vi "ziModGetCounterData.vi"(8 "Error In":errorcluster, 10 "ModResults":T3, 11 "ModHandle In":T6 {"ModHandle" format="0x%08x"; "Conn" format="0x%08x"}) -> (0 "Error Out":errorcluster, 2 "ModCntData":T2[](array[typedef]), 3 "ModHandle Out":T6 {"ModHandle" format="0x%08x"; "Conn" format="0x%08x"})   [LabVIEW 2009, in "Zurich Instruments LabOne.lvlib"]
doc: "Use this vi to get Counter Data from a ModResult returned from ziModGetNextNode.vi. It returns an array of Counter Data."
uses:
  <instrlib>/Zurich Instruments LabOne/Zurich Instruments LabOne.lvlib
  <instrlib>/Zurich Instruments LabOne/Public/Modules/ziTypeModHandle.ctl
  <instrlib>/Zurich Instruments LabOne/Public/Modules/ziTypeModResults.ctl
  <instrlib>/Zurich Instruments LabOne/Public/Data/ziTypePollType.ctl
  <instrlib>/Zurich Instruments LabOne/Public/Modules/ziTypeModGenericHeader.ctl
  <instrlib>/Zurich Instruments LabOne/Public/Data/ziTypeCounterSample.ctl
  <instrlib>/Zurich Instruments LabOne/Public/Data/ziTypeCounterSampleGrid.ctl
  <instrlib>/Zurich Instruments LabOne/Private/ziLV32.dll
panel:
  out "ModCntDataGrid":T1[](array[typedef])
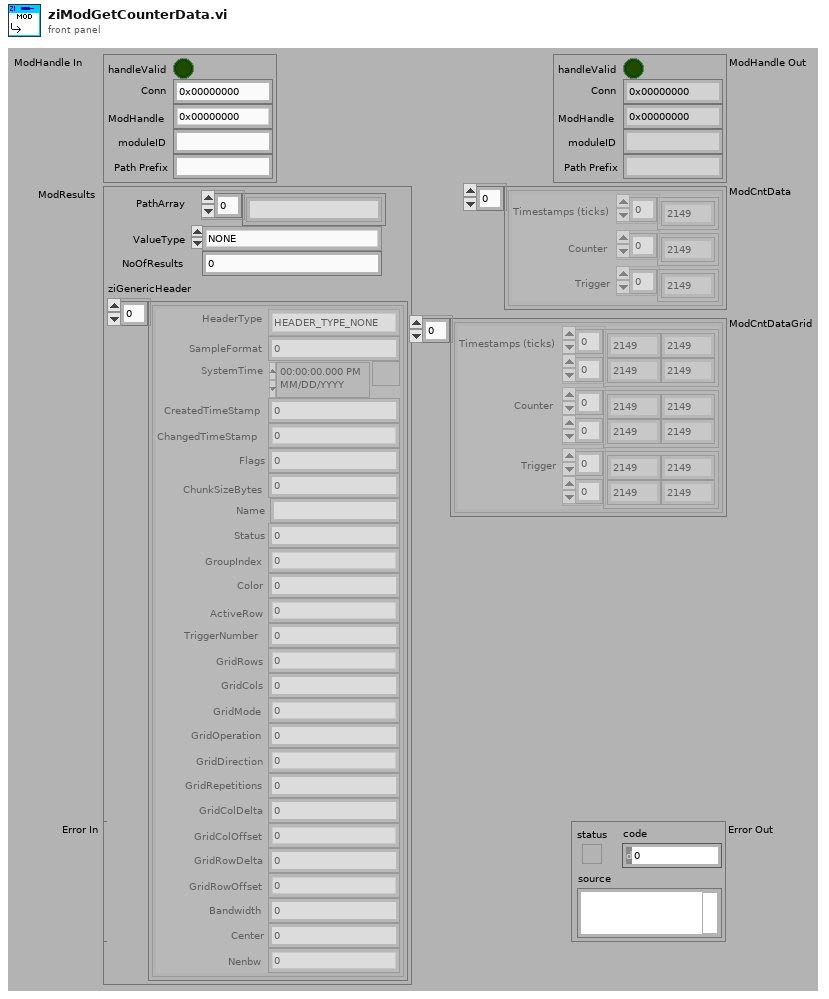
[diagram p1: front panel]
types:
  T1 = typedef "Zurich Instruments LabOne.lvlib/ziTypeCounterSampleGrid.ctl" = cluster{"Timestamps (ticks)":u64[][], "Counter":i32[][], "Trigger":u32[][]}
  T2 = typedef "Zurich Instruments LabOne.lvlib/ziTypeCounterSample.ctl" = cluster{"Timestamps (ticks)":u64[], "Counter":i32[], "Trigger":u32[]}
  T3 = typedef "Zurich Instruments LabOne.lvlib/ziTypeModResults.ctl" = cluster{"PathArray":string[], "ValueType":T4, "NoOfResults":u64, "ziGenericHeader":T5[]}
  T4 = typedef "Zurich Instruments LabOne.lvlib/ziTypePollType.ctl" = enum16{"NONE", "DOUBLE_DATA", "INTEGER_DATA", "DEMOD_SAMPLE", "SCOPE_WAVE_HF2", "AUXIN_SAMPLE", "DIO_SAMPLE", "BYTE_ARRAY", "PWA_WAVE", "9", "10", "11", "12", "13", "14", "15", "TREE_CHANGE_DEPRI", "17", "ERROR", "19", "20", "21", "22", "23", "24", "25", "26", "27", "28", "29", "30", "31", "DOUBLE_DATA_TS", "INTEGER_DATA_TS", "34", "SCOPE_WAVE", "SCOPE_WAVE_EX", "37", "BYTE_ARRAY_TS", "39", "40", "41", "42", "43", "44", "45", "CNT_DATA", "47", "TREE_CHANGE", "49", "50", "51", "52", "53", "54", "55", "56", "57", "58", "59", "60", "61", "62", "63", "SWEEPER_DATA", "SPECTRUM_DATA", "ADVISOR_DATA", "VECTOR_DATA", "IMP_DATA"}
  T5 = typedef "Zurich Instruments LabOne.lvlib/ziTypeModGenericHeader.ctl" = cluster{"HeaderType":enum8{"HEADER_TYPE_NONE", "HEADER_TYPE_SWTRIGGER", "HEADER_TYPE_SWEEPER"}, "SampleFormat":u8, "SystemTime":timestamp, "CreatedTimeStamp":u64, "ChangedTimeStamp":u64, "Flags":u32, "ChunkSizeBytes":u64, "Name":string, "Status":u32, "GroupIndex":u32, "Color":u32, "ActiveRow":u32, "TriggerNumber":u64, "GridRows":u32, "GridCols":u32, "GridMode":u32, "GridOperation":u32, "GridDirection":u32, "GridRepetitions":u32, "GridColDelta":dbl, "GridColOffset":dbl, "GridRowDelta":dbl, "GridRowOffset":dbl, "Bandwidth":dbl, "Center":dbl, "Nenbw":dbl}
  T6 = typedef "Zurich Instruments LabOne.lvlib/ziTypeModHandle.ctl" = cluster{"handleValid":bool, "Conn":u64, "ModHandle":u64, "moduleID":string, "Path Prefix":string}
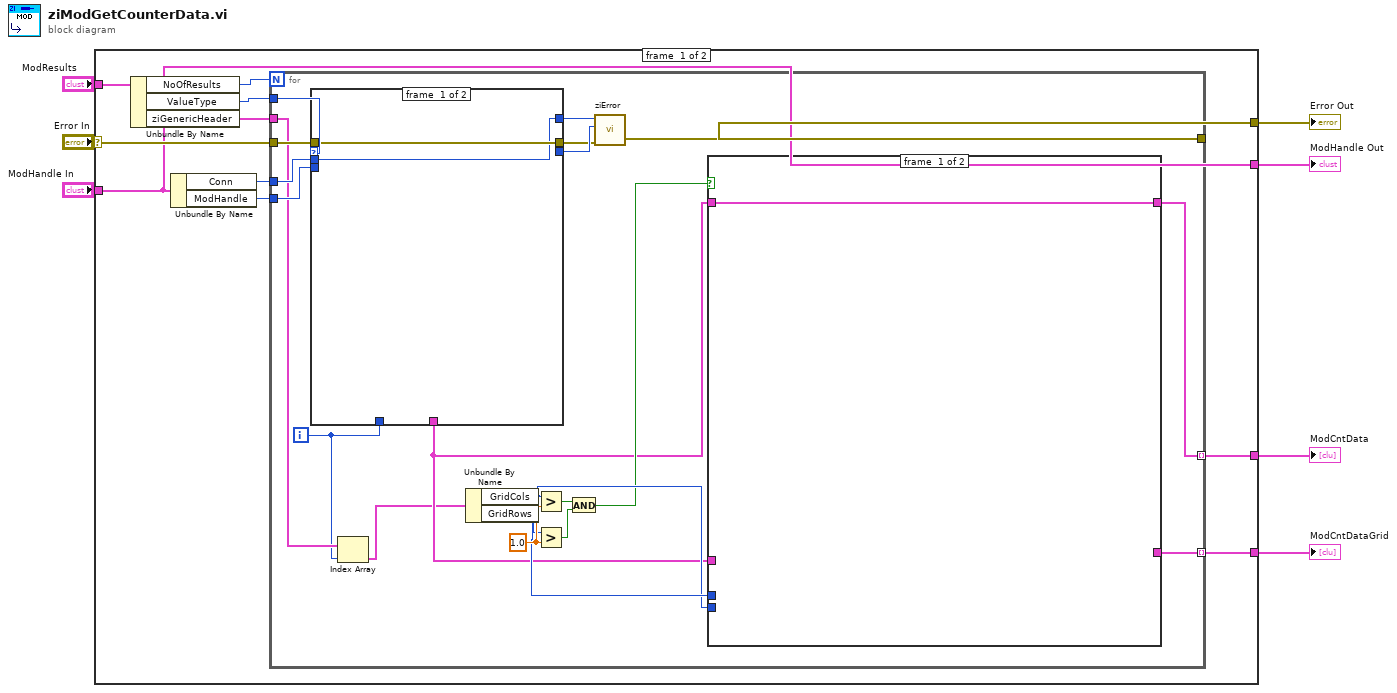
[diagram p0: block diagram]
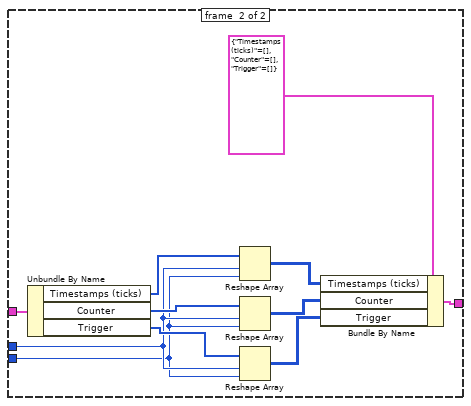
[diagram p2: hidden frame]
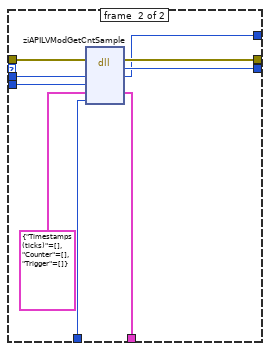
[diagram p3: hidden frame]
diagram:
  n1 = case shown="No Error" "Error In" {
    selector: "Error In" -> [w13 w62]
    tunnel: [w14 w62] -> w3
    tunnel: [w12 w63] -> w6
    tunnel: "ModHandle In" -> [w12 w63]
    tunnel: "ModResults" -> [w16 _]
    tunnel: [w10 _] -> w2
    tunnel: [w8 _] -> w1
    frame #0 {
      n2 = Unbundle By Name(w16) -> ("NoOfResults"=w15:u64, "ValueType"=w11:T4, "ziGenericHeader"=w9:T5[])
      n3 = Unbundle By Name(w12) -> ("Conn"=w18:u64, "ModHandle"=w17:u64)
      n4 = for {
        N: w15 -> [_]
        tunnel: w18 -> [w38]
        tunnel: w17 -> [w37]
        tunnel: [w36] -> w14
        tunnel: w13 -> [w33]
        tunnel: w11 -> [w32]
        tunnel: [w24] -> w10 mode=indexing
        tunnel: w9 -> [w21]
        tunnel: [w22] -> w8 mode=indexing
        i -> [w20]
        w28 = 1.0 ("y")
        n5 = case shown="\"CNT_DATA\"" w32 {
          tunnel: w38 -> [w51 w61]
          tunnel: w37 -> [_ w60]
          tunnel: w20 -> [_ w59]
          tunnel: [_ w58] -> w35
          tunnel: [w52 w57] -> w34
          tunnel: w33 -> [w52 w56]
          tunnel: [_ w55] -> w23
          tunnel: [w51 w54] -> w31
          frame #0 {
          }
          frame #1 {
            n6 = dll-call lib="C:/Program Files (x86)/National Instruments/LabVIEW 2009/instr.lib/Zurich Instruments LabOne/Private/ziLV*.*" fn="ziAPILVModGetCntSample"(error in=w56, "Conn"=w61, "ModHandle"=w60, "DEMODData"=T2 {"Timestamps (ticks)"=[], "Counter"=[], "Trigger"=[]}, "chunk_idx"=w59) -> (error out=w57:errorcluster, "return type"=w58:u32, "Conn"=w54:u64, "DEMODData"=w55:T2)  [unwired: 4 in, 1 out]
          }
        }
        n7 = Index Array(array=w21, index=w20) -> (element=w19:T5)
        n8 = Unbundle By Name(w19) -> ("GridCols"=w26:u32, "GridRows"=w27:u32)
        n9 = Greater?(x=w26, y=w28) -> (0:w30:bool)
        n10 = Greater?(x=w27, y=w28) -> (0:w29:bool)
        n11 = And(x=w30, y=w29) -> (x .and. y?=w25:bool)
        n12 = call <instrlib>:"ziError.vi"("Conn"=w31, "ziErrorCode"=w35, "Error In"=w34) -> ("Error Out"=w36:errorcluster)  [unwired: 2 in, 1 out]
        n13 = case shown="True" w25 {
          tunnel: w23 -> [_ w50]
          tunnel: w23 -> [w39 _]
          tunnel: [w39 _] -> w24
          tunnel: w27 -> [_ w46]
          tunnel: w26 -> [_ w43]
          tunnel: [_ w45] -> w22
          frame #0 {
          }
          frame #1 {
            n14 = Unbundle By Name(w50) -> ("Timestamps (ticks)"=w49:u64[], "Counter"=w48:i32[], "Trigger"=w47:u32[])
            n15 = Reshape Array(w49, w46, w43) -> (w42:u64[][])
            n16 = Reshape Array(w48, w46, w43) -> (w41:i32[][])
            n17 = Reshape Array(w47, w46, w43) -> (w40:u32[][])
            n18 = Bundle By Name(cluster=T1 {"Timestamps (ticks)"=[], "Counter"=[], "Trigger"=[]} ("Imp Sample"), "Timestamps (ticks)"=w42, "Counter"=w41, "Trigger"=w40) -> (w45:T1)
          }
        }
      }
    }
    frame #1 {
    }
  }
  "Error Out" <- w3
  "ModHandle Out" <- w6
  "ModCntData" <- w2
  "ModCntDataGrid" <- w1
